vi "油门.vi"() -> ()   [LabVIEW 2022 SP3]
panel:
  in  "停止":bool
  out "油量指示灯":bool
  out "显示面板":T1 {"油量（升）" scale=0.0..100.0; "转速（转/秒）" scale=0.0..10000.0; "时速（公里/小时）" scale=0.0..200.0}
  in  "控制面板":T2 {"挡位" scale=0.0..5.0; "油门" scale=0.0..100.0}
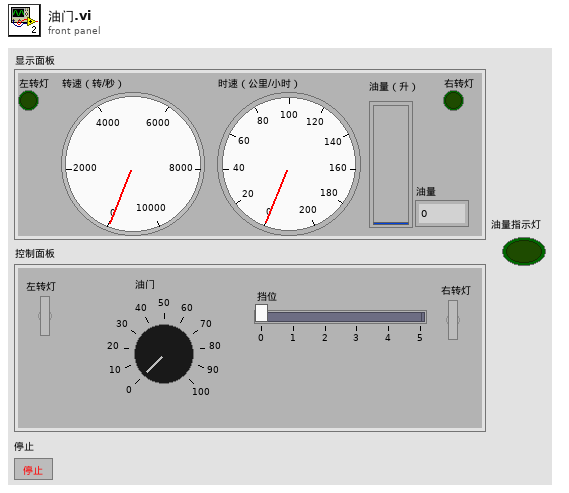
[diagram p1: front panel]
types:
  T1 = cluster{"左转灯":bool, "右转灯":bool, "转速（转/秒）":dbl, "时速（公里/小时）":dbl, "油量（升）":dbl, "油量":dbl}
  T2 = cluster{"左转灯":bool, "右转灯":bool, "油门":dbl, "挡位":dbl}
  T3 = cluster{"左转灯":bool, "右转灯":bool, dbl, dbl, i32, i32}
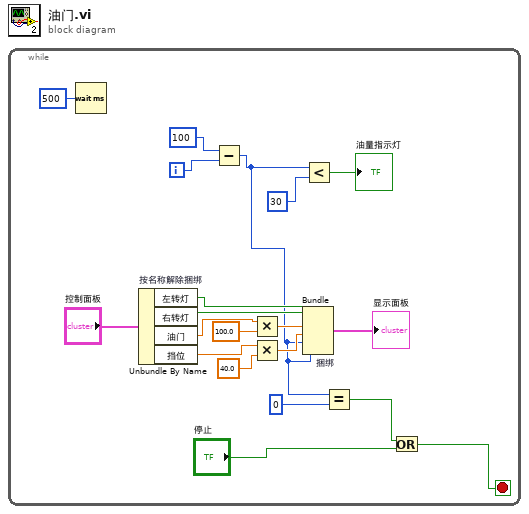
[diagram p0: block diagram]
diagram:
  n1 = while {
    i -> [w10]
    stop <- w2 stop-if-true
    n2 = Wait (ms)(milliseconds to wait=u32 500 ("等待时间（毫秒）")) -> ()  [unwired: 1 out]
    n3 = Unbundle By Name "按名称解除捆绑"("控制面板") -> ("左转灯"=w19:bool, "右转灯"=w18:bool, "油门"=w17:dbl, "挡位"=w13:dbl)
    n4 = Subtract(x=100, y=w10) -> (x-y=w5:i32)
    n5 = Multiply(x=w17, y=100.0) -> (x*y=w16:dbl)
    n6 = Multiply(x=w13, y=40.0) -> (x*y=w14:dbl)
    n7 = Bundle "捆绑"("左转灯"=w19, "右转灯"=w18, w16, w14, w5, w5) -> (→"显示面板":T3)  [unwired: 1 in]
    n8 = Less?(x=w5, y=30) -> (x < y?=→"油量指示灯":bool)
    n9 = Equal?(x=w5, y=0) -> (x = y?=w3:bool)
    n10 = Or(x=w3, y="停止") -> (x .or. y?=w2:bool)
  }
